vi "sequences to string.vi"(11 "sequence definitions":T1[](array[typedef])) -> (3 "string":string)   [LabVIEW 2014, in "Simple Sequencer TBM configuration.lvclass"]
uses:
  Simple Sequencer TBM configuration.lvclass
  sequence definition.ctl
  sequencer parent classes/action configuration parent/action configuration.lvclass
  <vilib>/NI/Configuration Framework/serializable configuration/NISE_CEF_serializable configuration.lvclass
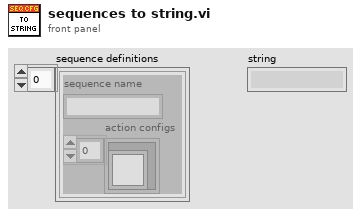
[diagram p1: front panel]
types:
  T1 = typedef "Simple Sequencer TBM configuration.lvclass/sequence definition.ctl" = cluster{"sequence name":string, "action configs":refnum<class "action configuration.lvclass">[]}
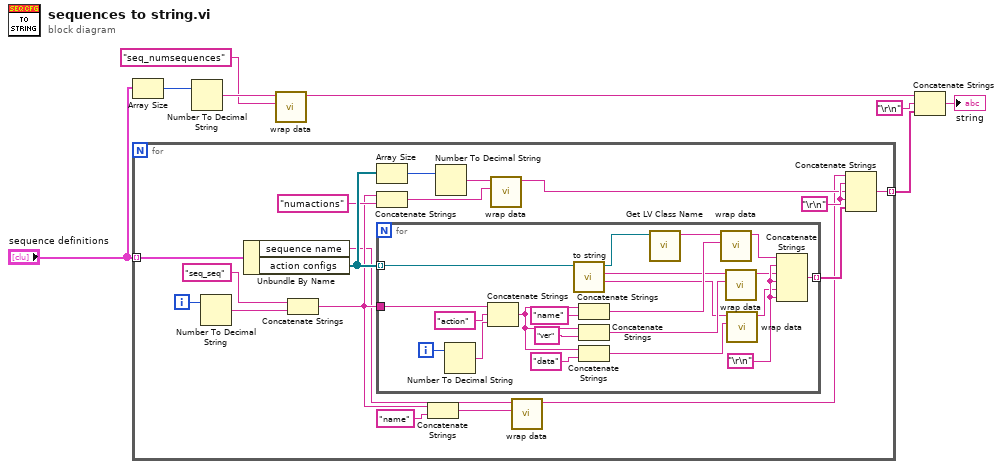
[diagram p0: block diagram]
diagram:
  n1 = Array Size(array="sequence definitions") -> (size(s)=w7:i32)
  n2 = for {
    tunnel: "sequence definitions" -> [w26] mode=indexing
    tunnel: [w15] -> w6 mode=indexing
    i -> [w25]
    w16 = "\r\n"
    n3 = Number To Decimal String(number=w25) -> (decimal integer string=w23:string)  [unwired: 1 in]
    n4 = Unbundle By Name(w26) -> ("sequence name"=w11:string, "action configs"=w21:refnum<class "action configuration.lvclass">[])
    n5 = Concatenate Strings("seq_seq" ("identifier"), w23) -> (w18:string)
    n6 = Array Size(array=w21) -> (size(s)=w22:i32)
    n7 = Concatenate Strings(w18, "numactions" ("string")) -> (w13:string)
    n8 = for {
      tunnel: w21 -> [w47] mode=indexing
      tunnel: w18 -> [w44]
      tunnel: [w45] -> w17 mode=indexing
      i -> [w46]
      w38 = "\r\n"
      n9 = Number To Decimal String(number=w46) -> (decimal integer string=w42:string)  [unwired: 1 in]
      n10 = Concatenate Strings(w44, "action" ("string"), w42) -> (w37:string)
      n11 = call-dynamic "to string.vi"("configuration in"=w47) -> ("data"=w28:string, "version"=w31:string, "configuration out"=w39:refnum<class "action configuration.lvclass">)  [unwired: 7 in, 1 out]
      n12 = Concatenate Strings(w37, "name" ("string")) -> (w33:string)
      n13 = Concatenate Strings(w37, "ver" ("string")) -> (w30:string)
      n14 = Concatenate Strings(w37, "data" ("string")) -> (w27:string)
      n15 = call <vilib>:"Get LV Class Name.vi"("object"=w39) -> ("class name"=w34:string)  [unwired: 9 in, 1 out]
      n16 = call <vilib>:"wrap data.vi"("identifier"=w33, "data to wrap"=w34) -> ("wrapped data"=w35:string)  [unwired: 9 in]
      n17 = call <vilib>:"wrap data.vi"("identifier"=w30, "data to wrap"=w31) -> ("wrapped data"=w32:string)  [unwired: 9 in]
      n18 = call <vilib>:"wrap data.vi"("identifier"=w27, "data to wrap"=w28) -> ("wrapped data"=w29:string)  [unwired: 9 in]
      n19 = Concatenate Strings(w35, w38, w32, w38, w29, w38) -> (w45:string)
    }
    n20 = Concatenate Strings(w18, "name" ("string")) -> (w9:string)
    n21 = Number To Decimal String(number=w22) -> (decimal integer string=w14:string)  [unwired: 1 in]
    n22 = call <vilib>:"wrap data.vi"("identifier"=w13, "data to wrap"=w14) -> ("wrapped data"=w12:string)  [unwired: 9 in]
    n23 = call <vilib>:"wrap data.vi"("identifier"=w9, "data to wrap"=w11) -> ("wrapped data"=w10:string)  [unwired: 9 in]
    n24 = Concatenate Strings(w10, w16, w12, w16, w17) -> (w15:string)
  }
  n25 = Number To Decimal String(number=w7) -> (decimal integer string=w3:string)  [unwired: 1 in]
  n26 = call <vilib>:"wrap data.vi"("identifier"="seq_numsequences", "data to wrap"=w3) -> ("wrapped data"=w2:string)  [unwired: 9 in]
  n27 = Concatenate Strings(w2, "\r\n", w6) -> (→"string":string)
